vi "Create channel.vi"(8 "error in (no error)":errorcluster, 10 "Lines":T1[](array[typedef])=[1] items=["DIO1...8"=1, "DIO9...16"=2, "DIO17...24"=3, "DIO25...32"=4], 11 "Connection ID":i32=-1) -> (0 "error out":errorcluster, 3 "MicroDAQ.lvlib:Digital Input.lvclass":refnum<class "Digital Input.lvclass">)   [LabVIEW 2009, in "MicroDAQ.lvlib" / "Digital Input.lvclass"]
uses:
  <instrlib>/MicroDAQ/Channel/Digital Input/Digital Input.lvclass
  <instrlib>/MicroDAQ/Tools/Digital IO channels.ctl
  <instrlib>/MicroDAQ/Channel/Digital Input/Digital Input.lvclass/Digital Input.ctl
  <instrlib>/MicroDAQ/Mlink library wraper/mlink.lvlib
  <instrlib>/MicroDAQ/Tools/DIO set direction argument.ctl
  <instrlib>/MicroDAQ/MicroDAQ.lvlib
  <instrlib>/MicroDAQ/Channel/Channel.lvclass
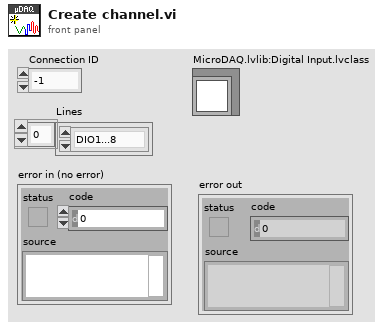
[diagram p1: front panel]
types:
  T1 = typedef "MicroDAQ.lvlib/Digital IO channels.ctl" = u8
  T2 = typedef "MicroDAQ.lvlib/DIO set direction argument.ctl" = enum8{"Input", "Output"}
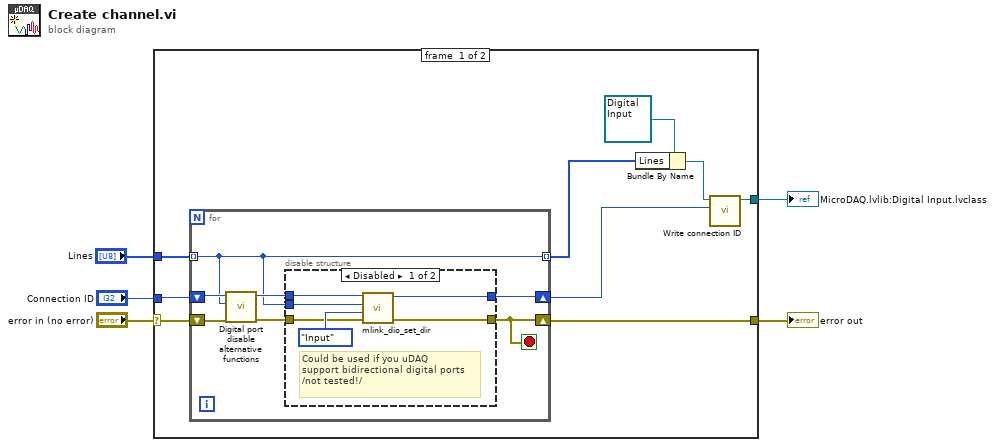
[diagram p0: block diagram]
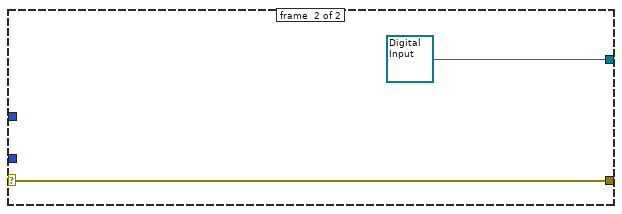
[diagram p3: hidden frame]
diagram:
  n1 = case shown="No Error" "error in (no error)" {
    selector: "error in (no error)" -> [w13 w30]
    tunnel: "Connection ID" -> [w14 _]
    tunnel: "Lines" -> [w12 _]
    tunnel: [w11 w30] -> w3
    tunnel: [w9 refnum<class "Digital Input.lvclass"> refnum ("Task out")] -> w2
    frame #0 {
      n2 = for {
        tunnel: w12 -> [w15] mode=indexing
        shift-right: [w18] -> w10
        shift-left: w14 -> [w16]
        shift-right: [w17] -> w11
        shift-left: w13 -> [w21]
        tunnel: [w15] -> w6 mode=indexing
        stop <- w17 stop-if-true
        n3 = call <instrlib>:"Digital port disable alternative functions.vi"("error in (no error)"=w21, "Lines"=w15, "Connection ID"=w16) -> ("error out"=w19:errorcluster, "connection ID out"=w20:i32)  [unwired: 7 in]
        n4 = disable-structure shown="Disabled" {
          disable-tunnel: w20 -> [w27 w29]
          disable-tunnel: w19 -> [w25 w28]
          disable-tunnel: [w24 w29] -> w18
          disable-tunnel: [w23 w28] -> w17
          disable-tunnel: w15 -> [w22 _]
          frame #0 {
            # "Could be used if you uDAQ\nsupport bidirectional digital ports\n/not tested!/"
            n5 = call <instrlib>:"mlink_dio_set_dir.vi"("error in (no error)"=w25, "direction"=DIO_set_direction_argument."Input", "bank"=w22, "connection ID"=w27) -> ("error out"=w23:errorcluster, "connection ID out"=w24:i32)  [unwired: 6 in]
          }
          frame #1 {
          }
        }
      }
      n6 = Bundle By Name(cluster=refnum<class "Digital Input.lvclass"> refnum ("MicroDAQ.lvlib:Digital Input.lvclass"), "Lines"=w6) -> (w7:refnum<class "Digital Input.lvclass">)
      n7 = call <instrlib>:"Write connection ID.vi"("connection ID"=w10, "Task in"=w7) -> ("Task out"=w9:refnum<class "Digital Input.lvclass">)  [unwired: 9 in]
    }
    frame #1 {
    }
  }
  "error out" <- w3
  "MicroDAQ.lvlib:Digital Input.lvclass" <- w2
